vi "MinerSubmitJob.vi"(3 "error in (no error)":errorcluster, 4 "JobDoneString":string, 5 "connection ID":refnum<k5>) -> (0 "error out":errorcluster, 1 "FeedBack":string="2.4", 2 "connection ID out":refnum<k5>)   [LabVIEW 2014]
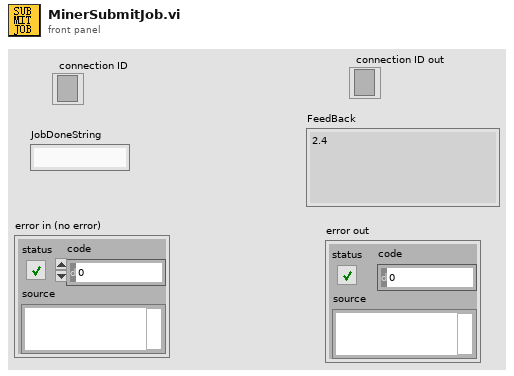
[diagram p1: front panel]
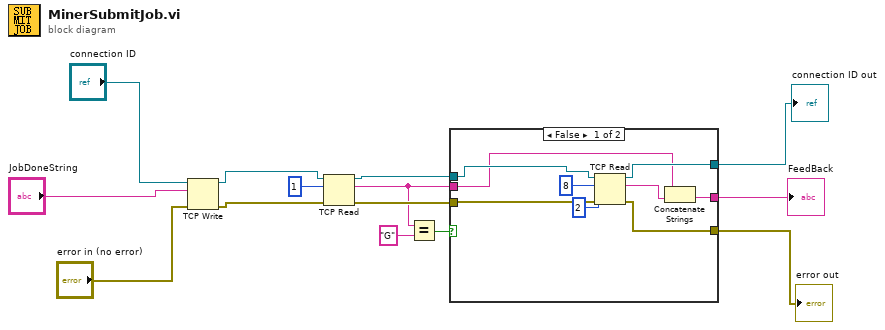
[diagram p0: block diagram]
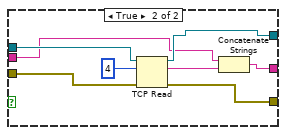
[diagram p2: hidden frame]
diagram:
  n1 = TCP Write(connection ID="connection ID", data in="JobDoneString", error in (no error)="error in (no error)") -> (connection ID out=w11:refnum<k5>, error out=w10:errorcluster)  [unwired: 1 in, 1 out]
  n2 = TCP Read(connection ID=w11, bytes to read=1 ("读取的字节"), error in (no error)=w10) -> (connection ID out=w6:refnum<k5>, data out=w1:string, error out=w5:errorcluster)  [unwired: 2 in]
  n3 = Equal?(x=w1, y="G") -> (x = y?=w7:bool)
  n4 = case shown="False" w7 {
    tunnel: w6 -> [w21 w30]
    tunnel: w5 -> [w22 w29]
    tunnel: [w17 w27] -> w4
    tunnel: [w19 w26] -> w3
    tunnel: [w18 w25] -> w2
    tunnel: w1 -> [w15 w24]
    frame False {
      n5 = TCP Read(connection ID=w21, bytes to read=8 ("读取的字节"), error in (no error)=w22, 9:2 ("timeout ms (25000)")) -> (connection ID out=w19:refnum<k5>, data out=w16:string, error out=w18:errorcluster)  [unwired: 1 in]
      n6 = Concatenate Strings(w15, w16) -> (w17:string)
    }
    frame True {
      n7 = TCP Read(connection ID=w30, bytes to read=4 ("读取的字节"), error in (no error)=w29) -> (connection ID out=w26:refnum<k5>, data out=w28:string, error out=w25:errorcluster)  [unwired: 2 in]
      n8 = Concatenate Strings(w24, w28) -> (w27:string)
    }
  }
  "FeedBack" <- w4
  "error out" <- w2
  "connection ID out" <- w3
